vi "Matches.vi"() -> ()   [LabVIEW 2017]
panel:
  in  "OK":bool
  out "HowTo":string
  # "Histórico"
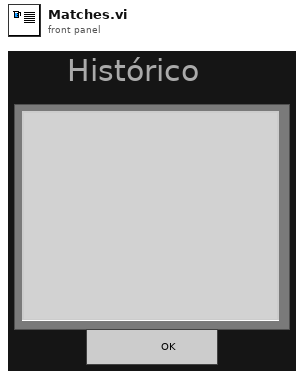
[diagram p1: front panel]
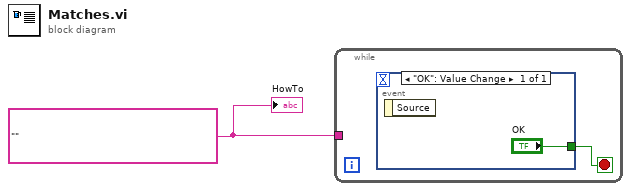
[diagram p0: block diagram]
diagram:
  w1 = ""
  n1 = while {
    tunnel: w1 -> [_]
    stop <- w2 stop-if-true
    n2 = event shown="[0] \"OK\": Value Change" {
      selector: _ -> [_]
      dyn-events: _ -> [_]
      timeout: _ -> [_]
      tunnel: ["OK"] -> w2
      event "OK": Value Change {
        n3 = event-data() -> ()  [unwired: 1 in, 1 out]
      }
    }
  }
  "HowTo" <- w1
